vi "Prox_StateMachine.vi"(8 "error in (no error)":errorcluster) -> (0 "error out":errorcluster, 3 "aReaderName":string)   [LabVIEW 2019]
uses:
  WinSCard.dll
panel:
  out "status":string
  out "time":string
  out "pbRecvBuffer":string
  out "bATR (Answer to Reset)":string
  out "Free Memory":i32
  out "transmit":i32 format="%x"
  out "Disconnect Return":u32 format="%x"
  out "Release Context Return":u32 format="%x"
  out "Reader Return":i32 format="%x"
  out "Establish Return":u32 format="%x"
  out "Card Connect Return":u32 format="%x"
  out "Card Status Return":u32 format="%x"
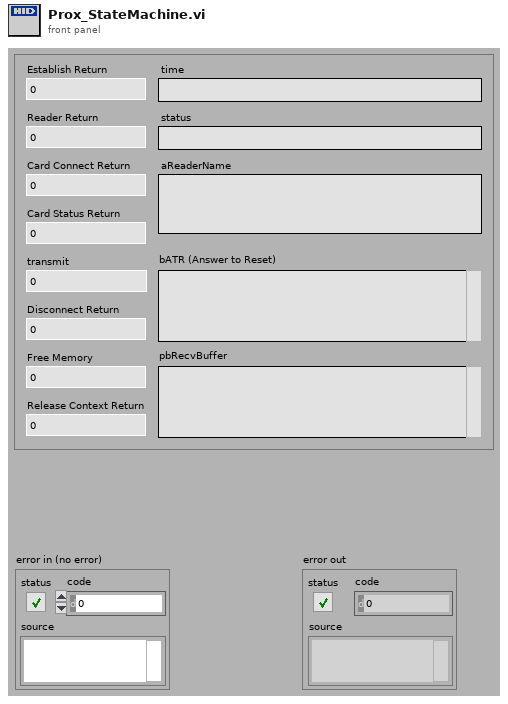
[diagram p1: front panel]
types:
  T1 = enum32{"Invalid", "Standard", "Closed", "Hidden", "Minimized", "Maximized"}
  T2 = enum32{"invalid app kind", "Development System", "Run Time System", "Student Edition", "Embedded LabVIEW", "Evaluation", "Custom"}
  T3 = enum16{"initialize", "reader present", "card connected", "card disconnected", "shutdown"}
  T4 = cluster{"Core":cluster{"Current VI Reference":refnum<vi>, "Close Panel on Exit?":bool}, "hContextHandle":u32, "hCardHandle":u32, "szReader":string, "status":enum16{"initialize", "reader present", "card connected", "card disconnected", "shutdown"}}
  T5 = cluster{"Current VI Reference":refnum<vi>, "Close Panel on Exit?":bool}
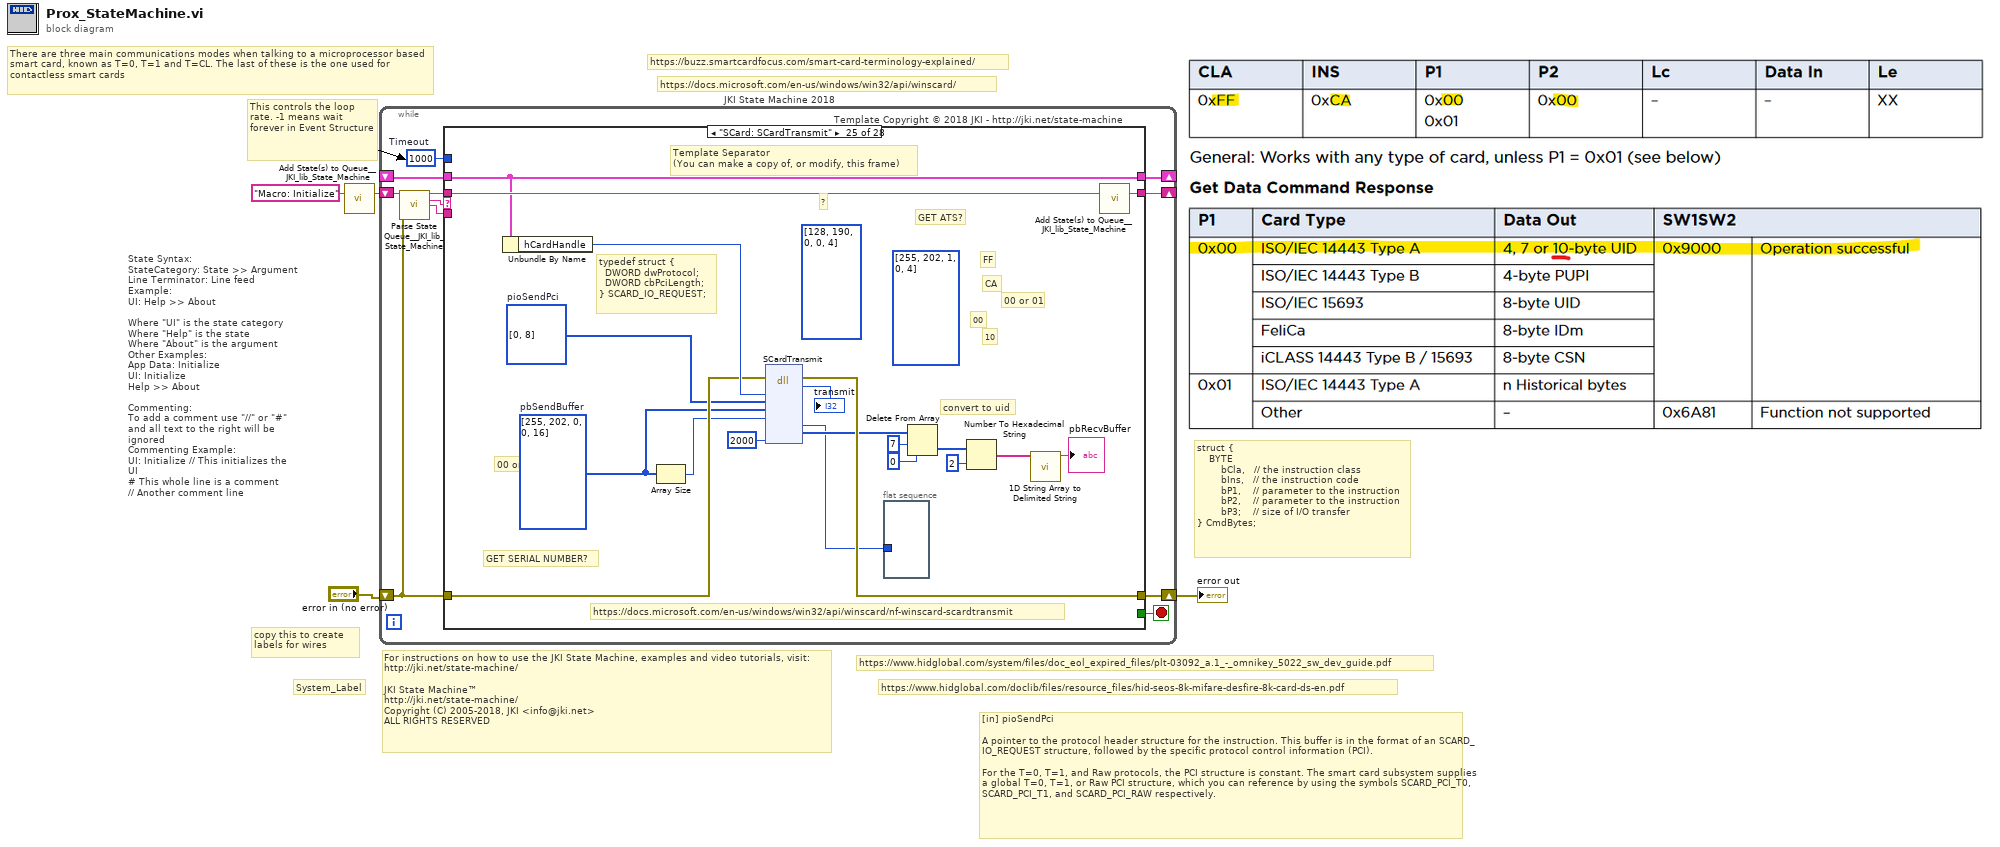
[diagram p0: block diagram]
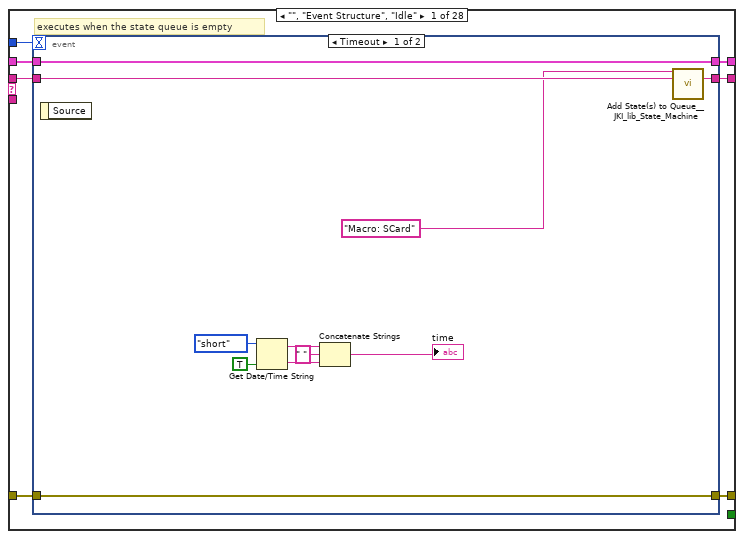
[diagram p2: hidden frame]
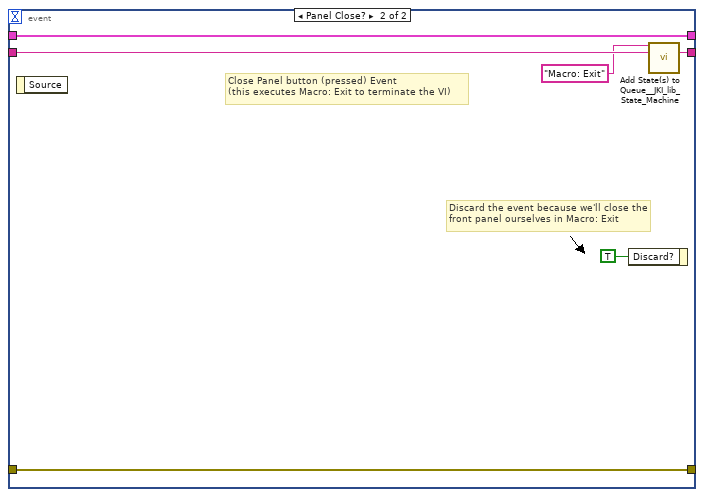
[diagram p3: hidden frame]
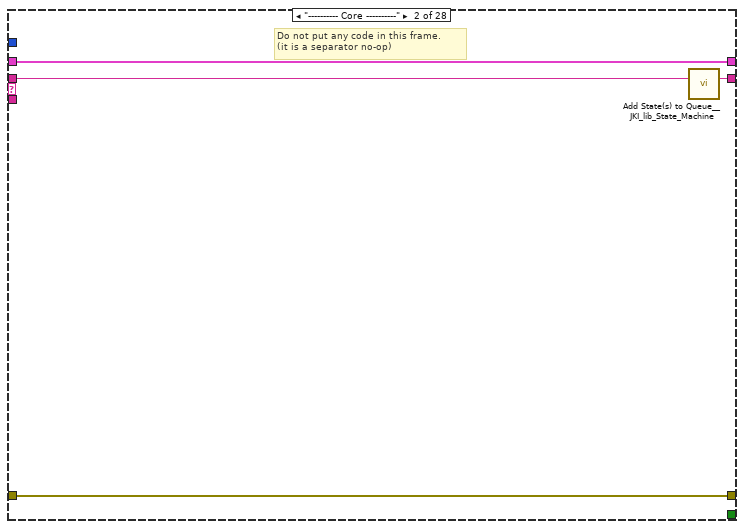
[diagram p4: hidden frame]
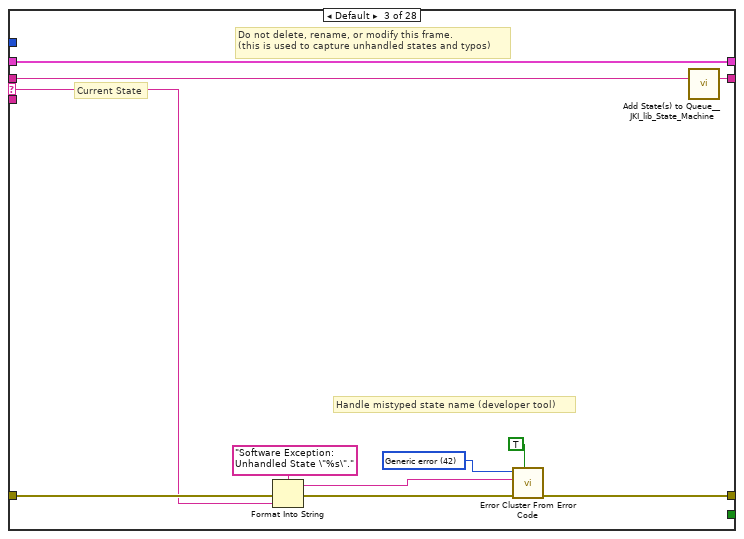
[diagram p5: hidden frame]
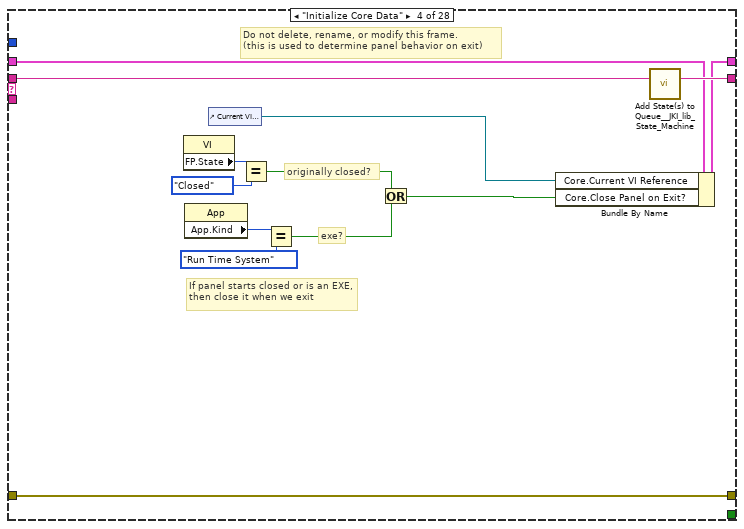
[diagram p6: hidden frame]
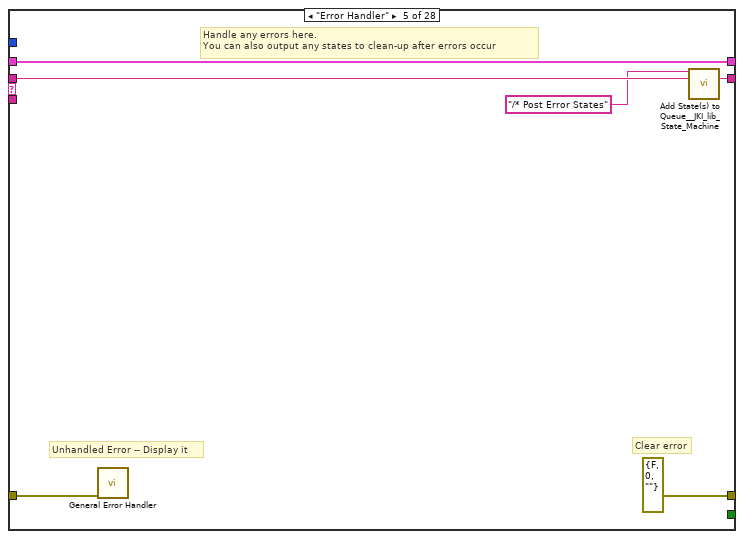
[diagram p7: hidden frame]
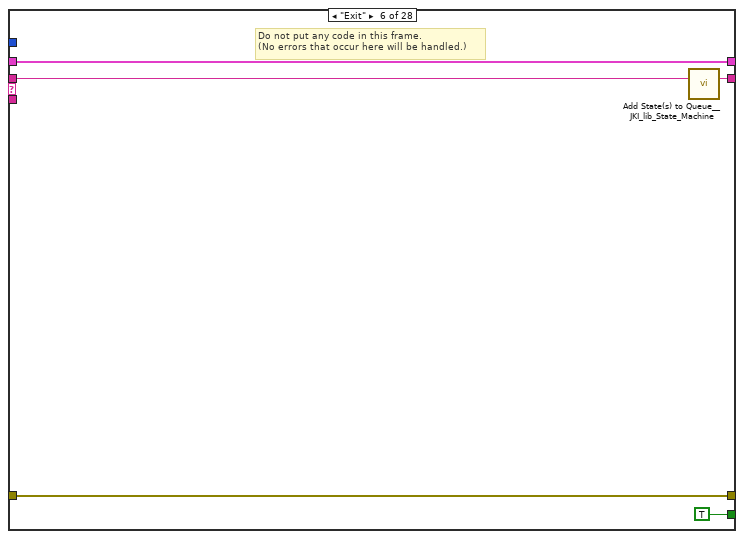
[diagram p8: hidden frame]
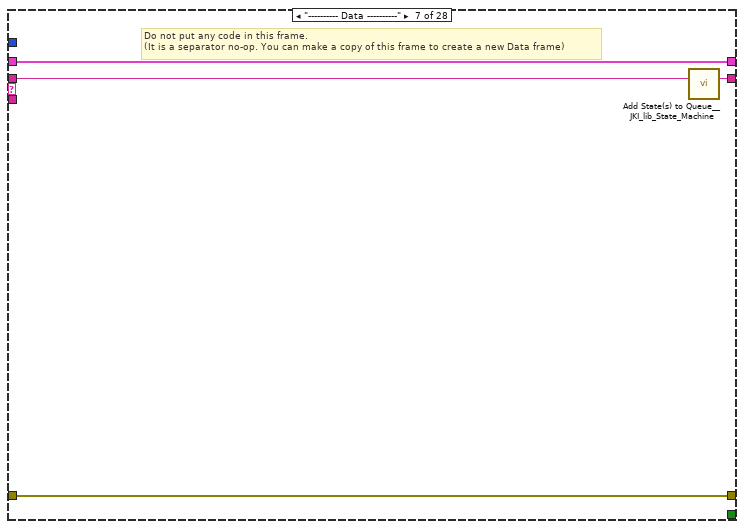
[diagram p9: hidden frame]
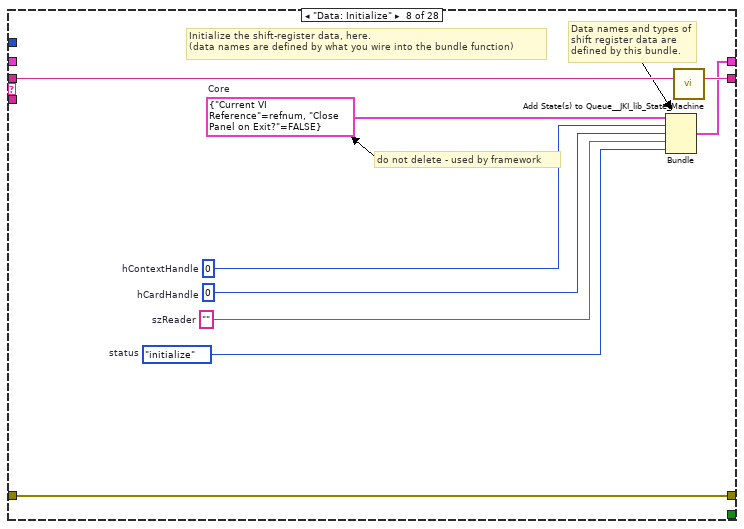
[diagram p10: hidden frame]
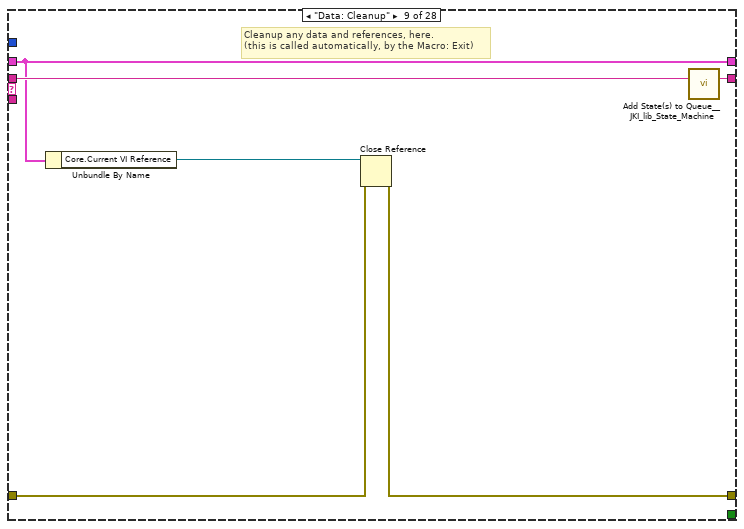
[diagram p11: hidden frame]
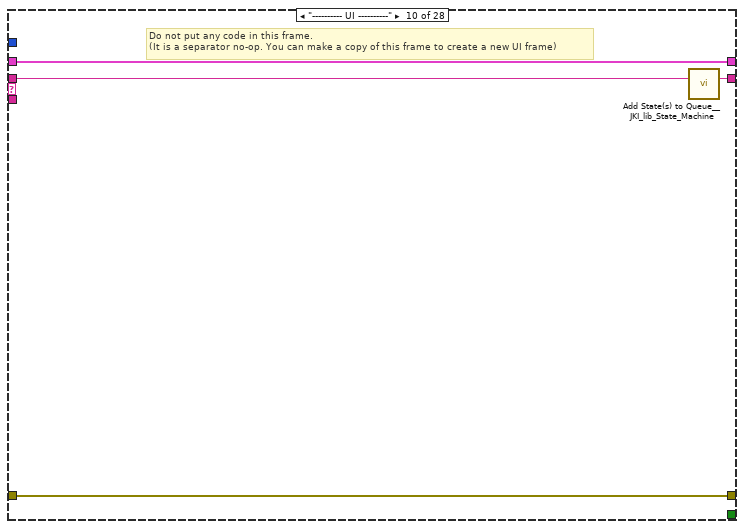
[diagram p12: hidden frame]
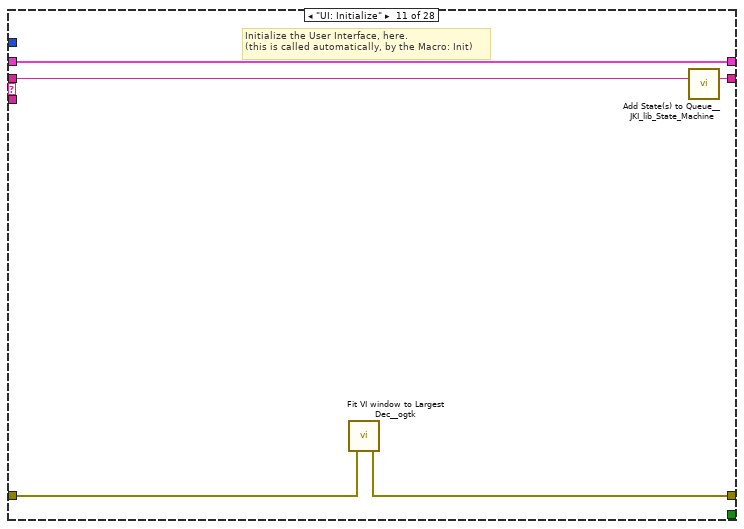
[diagram p13: hidden frame]
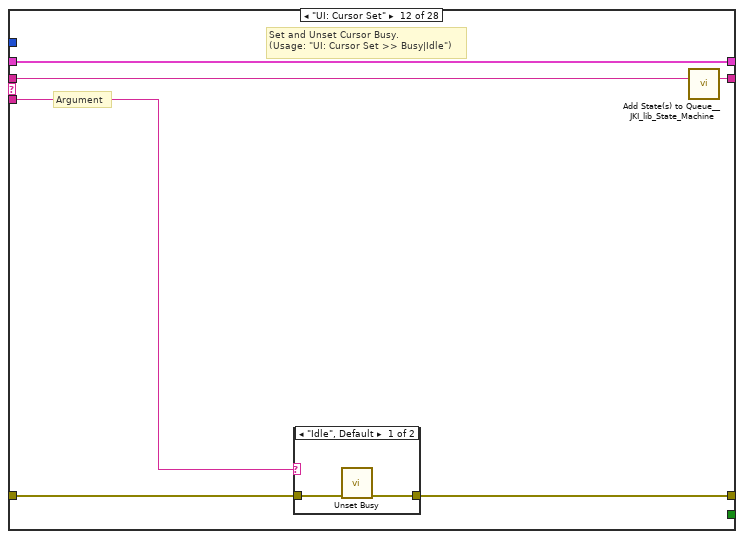
[diagram p14: hidden frame]
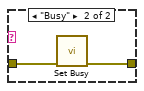
[diagram p15: hidden frame]
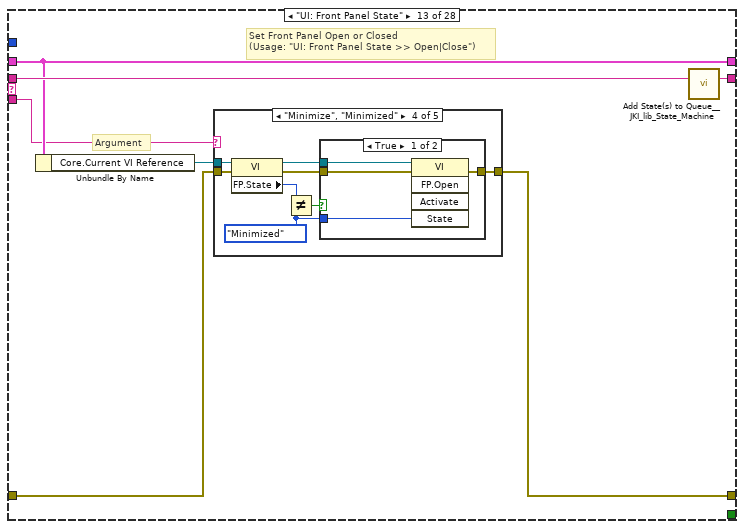
[diagram p16: hidden frame]
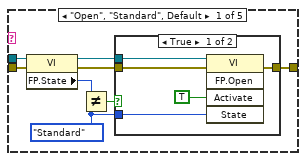
[diagram p17: hidden frame]
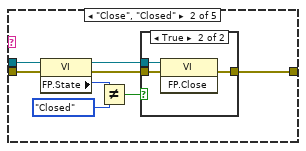
[diagram p19: hidden frame]
diagram:
  # "https://www.hidglobal.com/doclib/files/resource_files/hid-seos-8k-mifare-desfire-8k-card-ds-en.pdf"
  # "https://www.hidglobal.com/system/files/doc_eol_expired_files/plt-03092_a.1_-_omnikey_5022_sw_dev_guide.pdf"
  # "struct {\n    BYTE\n        bCla,   // the instruction class\n        bIns,   // the instruction code \n        bP1,    // parameter to the instruction\n        bP2,    // parameter to the instruction\n        bP3;    // size of I/O transfer\n} CmdBytes;"
  # "There are three main communications modes when talking to a microprocessor based smart card, known as T=0, T=1 and T=CL. The last of these is the one used for contactless smart cards"
  # "https://docs.microsoft.com/en-us/windows/win32/api/winscard/"
  # "For instructions on how to use the JKI State Machine, examples and video tutorials, visit:\nhttp://jki.net/state-machine/\n\nJKI State Machine™\nhttp://jki.net/state-machine/\nCopyright (C) 2005-2018, JKI <info@jki.net>\nALL RIGHTS RESERVED"
  # "State Syntax:\nStateCategory: State >> Argument\nLine Terminator: Line feed\nExample:\nUI: Help >> About\n\nWhere \"UI\" is the state category\nWhere \"Help\" is the state\nWhere \"About\" is the argument\nOther Examples:\nApp Data: Initialize\nUI: Initialize\nHelp >> About\n\nCommenting:\nTo add a comment use \"//\" or \"#\" and all text to the right will be ignored\nCommenting Example:\nUI: Initialize // This initializes the UI\n# This whole line is a comment\n// Another comment line"
  # "copy this to create labels for wires"
  # "This controls the loop rate. -1 means wait forever in Event Structure"
  # "System_Label"
  # "https://buzz.smartcardfocus.com/smart-card-terminology-explained/"
  # "[in] pioSendPci\n\nA pointer to the protocol header structure for the instruction. This buffer is in the format of an SCARD_IO_REQUEST structure, followed by the specific protocol control information (PCI).\n\nFor the T=0, T=1, and Raw protocols, the PCI structure is constant. The smart card subsystem supplies a global T=0, T=1, or Raw PCI structure, which you can reference by using the symbols SCARD_PCI_T0, SCARD_PCI_T1, and SCARD_PCI_RAW respectively."
  n1 = call <vilib>:"Add State(s) to Queue__JKI_lib_State_Machine.vi"("State(s) in (\"\")"="Macro: Initialize") -> ("States Out"=w4:string)  [unwired: 14 in]
  n2 = while "JKI State Machine 2018" {
    shift-right: [w8] -> _
    shift-left: _ -> [w7]
    shift-right: [w11] -> w1
    shift-left: "error in (no error)" -> [w5]
    shift-right: [w10] -> _
    shift-left: w4 -> [w12]
    stop <- w9 stop-if-true
    w6 = 1000  # Timeout
    # "Template Copyright © 2018 JKI - http://jki.net/state-machine"
    n3 = call <vilib>:"Parse State Queue__JKI_lib_State_Machine.vi"("State Queue"=w12, "Error In (no error)"=w5) -> ("Remaining States"=w14:string, "Current State"=w15:string, "Arguments"=w13:string)  [unwired: 11 in]
    n4 = case shown="\"SCard: SCardTransmit\"" w15 {
      selector: w15 -> [_ _ w44 _ _ _ _ _ _ _ _ _ _ _ _ _ _ _ _ _ _ _ _ _ _ _ _ _]
      tunnel: w14 -> [w22 w43 w48 w67 w73 w78 w82 w91 w97 w101 w106 w112 w123 w194 w198 w203 w208 _ w221 w225 w235 w241 w258 w287 w306 w314 w322 w329]
      tunnel: w13 -> [_ _ _ _ _ _ _ _ _ _ _ w107 w117 _ _ _ _ _ _ _ _ _ _ _ _ _ _ _]
      tunnel: w7 -> [w20 w40 w46 w60 w70 w76 w79 _ w92 w98 w104 w110 w119 w191 w195 w200 w205 w209 w218 w222 w228 w244 w261 w282 w303 w309 w319 w327]
      tunnel: [w19 w41 w50 w64 errorcluster {"status"=FALSE, "code"=0, "source"=""} ("error out") w75 w80 w88 w93 w99 w103 w108 w120 w192 w196 w201 w206 w210 w219 w223 w231 w242 w267 w284 w301 w311 w317 w325] -> w11
      tunnel: w5 -> [w18 w41 w49 w64 w69 w75 w80 w88 w94 w99 w102 w109 w121 w192 w196 w201 w206 w210 w219 w223 w232 w249 w266 w283 w300 w310 w316 w324]
      tunnel: [w21 w42 w47 w66 w72 w77 w81 w90 w96 w100 w105 w111 w122 w193 w197 w202 w207 w211 w220 w224 w234 w252 w270 w286 w305 w313 w321 w328] -> w10
      tunnel: [_ _ _ _ _ TRUE _ _ _ _ _ _ _ _ _ _ _ _ _ _ _ _ _ _ _ _ _ _] -> w9
      tunnel: [w17 w40 w46 w65 w70 w76 w79 w89 w92 w98 w104 w110 w119 w191 w195 w200 w205 w209 w218 w222 w229 w245 w262 w282 w303 w309 w319 w327] -> w8
      tunnel: w6 -> [w16 _ _ _ _ _ _ _ _ _ _ _ _ _ _ _ _ _ _ _ _ _ _ _ _ _ _ _]
      frame "", "Event Structure", "Idle" {
        # "executes when the state queue is empty"
        n5 = event shown="[0] Timeout" {
          selector: _ -> [_ _]
          dyn-events: _ -> [_ _]
          timeout: w16 -> [_ _]
          tunnel: w22 -> [w33 w39]
          tunnel: [w32 w38] -> w21
          tunnel: w20 -> [w30 w36]
          tunnel: [w31 w37] -> w19
          tunnel: w18 -> [w31 w37]
          tunnel: [w30 w36] -> w17
          event Timeout {
            n6 = event-data() -> ()  [unwired: 1 in, 1 out]
            n7 = Get Date/Time String(date format (0)=enum16{"short", "long", "abbreviated"}."short", want seconds? (F)=TRUE) -> (date string=w28:string, time string=w27:string)  [unwired: 1 in]
            n8 = Concatenate Strings(w28, " " ("string"), w27) -> (→"time":string)
            n9 = call <vilib>:"Add State(s) to Queue__JKI_lib_State_Machine.vi"("State(s) in Front (\"\")"="Macro: SCard" ("State(s) in Front (\"\")"), "State(s) in (\"\")"=w33) -> ("States Out"=w32:string)  [unwired: 13 in]
          }
          event Panel Close? {
            # "Discard the event because we'll close the front panel ourselves in Macro: Exit"
            # "Close Panel button (pressed) Event\n(this executes Macro: Exit to terminate the VI)"
            n10 = event-data() -> ()  [unwired: 1 in, 1 out]
            n11 = event-data("Discard?"=TRUE) -> ()  [unwired: 1 in, 1 out]
            n12 = call <vilib>:"Add State(s) to Queue__JKI_lib_State_Machine.vi"("State(s) in Front (\"\")"="Macro: Exit", "State(s) in (\"\")"=w39) -> ("States Out"=w38:string)  [unwired: 13 in]
          }
        }
      }
      frame "---------- Core ----------" {
        # "Do not put any code in this frame.\n(it is a separator no-op)"
        n13 = call <vilib>:"Add State(s) to Queue__JKI_lib_State_Machine.vi"("State(s) in (\"\")"=w43) -> ("States Out"=w42:string)  [unwired: 14 in]
      }
      frame Default {
        w53 = 42 items=["No error", "Argument error", "Memory is full", "Out of zone", "End of file", "File already open", "Generic file I/O error", "File not found", "File permission error", "Disk is full", "Duplicate path", "Too many files open", "System feature not enabled", "Resource file not found", "Cannot add resource", "Resource not found", "Image not found", "Image memory error", "Pen does not exist", "Config type invalid", "Config token not found", "Config parse error", "Config memory error", "Bad external code format", "Bad external code offset", "External code not present", "Null window", "Destroy window error", "Null menu", "Print aborted", "Bad print record", "Print driver error", "Windows error during printing", "Memory error during printing", "Print dialog error", "Generic print error", "Invalid device refnum", "Device not found", "Device parameter error", "Device unit error", "Cannot open device", "Device call aborted", "Generic error", "Cancelled by user", "Object ID too low", "Object ID too high", "Object not in heap", "Unknown heap", "Unknown object (invalid DefProc)", "Unknown object (DefProc not in table)", "Message out of range", "Invalid (null) method", "Unknown message", "Manager call not supported", "Bad address", "Network operation in progress", "Network operation timed out", "Connection is busy", "Network attribute not supported", "Network error", "Address in use", "System out of memory", "Connection aborted", "Connection refused", "Not connected", "Already connected", "Connection closed", "Initialization error (interapplication manager)", "Bad occurrence", "Wait on unbound occurrence handler", "Occurrence queue overflow", "Datalog type conflict", "Unused", "Unrecognized type (interapplication manager)", "Memory corrupt", "Failed to make temporary DLL", "Old CIN version", "Drag socket not found", "Failed to load drop-object", "Failed to register OLE object", "Failed to release OLE object", "Format specifier type mismatch", "Unknown format specifier", "Too few format specifiers", "Too many format specifiers", "Scan failed", "Newer CIN version", "Error converting to variant", "Runtime menu error", "Password tampered", "Variant attribute not found", "Incompatible variant data type", "Event data is not available", "Event Store is not present", "Occurrence is not found", "Event Queue is not created", "Event info is not available", "Refnum passed is NULL", "Error retrieving Class GUID", "Error retrieving CoClass GUID", "Error retrieving TypeLib GUID.", "Bad built application magic bytes.", "Specific driver is different from the specific driver associated with the Logical Name.", "There is no session opened to the class driver.", "Max Error", "MAX - Error with config objects", "MAX - Error loading configuration", "MAX - Group not supported"]
        # "Current State"
        # "Do not delete, rename, or modify this frame.\n(this is used to capture unhandled states and typos)"
        # "Handle mistyped state name (developer tool)"
        n14 = Format Into String(format string="Software Exception: Unhandled State \"%s\"." ("message"), error in=w49, w44) -> (resulting string=w52:string, error out=w51:errorcluster)  [unwired: 1 in]
        n15 = call <vilib>:"Error Cluster From Error Code.vi"("show call chain? (False)"=TRUE, "error in (no error)"=w51, "error message (\"\")"=w52, "error code (0)"=w53) -> ("error out"=w50:errorcluster)  [unwired: 5 in]
        n16 = call <vilib>:"Add State(s) to Queue__JKI_lib_State_Machine.vi"("State(s) in (\"\")"=w48) -> ("States Out"=w47:string)  [unwired: 14 in]
      }
      frame "Initialize Core Data" {
        # "Do not delete, rename, or modify this frame.\n(this is used to determine panel behavior on exit)"
        # "originally closed?"
        # "exe?"
        # "If panel starts closed or is an EXE, then close it when we exit"
        n17 = property class="VI"() -> ("FP.State"=w57:T1)  [unwired: 2 in, 2 out]
        n18 = property class="App"() -> ("App.Kind"=w63:T2)  [unwired: 2 in, 2 out]
        n19 = control-ref of="Current VI Reference"() -> (w58:refnum<vi>)
        n20 = Equal?(x=w57, y=T1."Closed" ("Front Panel Window:State")) -> (x = y?=w55:bool)
        n21 = Equal?(x=w63, y=T2."Run Time System" ("Application:Kind")) -> (x = y?=w61:bool)
        n22 = Or(x=w55, y=w61) -> (x .or. y?=w59:bool)
        n23 = Bundle By Name(cluster=w60, "Core.Current VI Reference"=w58, "Core.Close Panel on Exit?"=w59) -> (w65:T4)
        n24 = call <vilib>:"Add State(s) to Queue__JKI_lib_State_Machine.vi"("State(s) in (\"\")"=w67) -> ("States Out"=w66:string)  [unwired: 14 in]
      }
      frame "Error Handler" {
        # "Unhandled Error -- Display it"
        # "Handle any errors here.\nYou can also output any states to clean-up after errors occur"
        # "Clear error"
        n25 = call <vilib>:"General Error Handler.vi"("error in (no error)"=w69) -> ()  [unwired: 10 in, 5 out]
        n26 = call <vilib>:"Add State(s) to Queue__JKI_lib_State_Machine.vi"("State(s) in Front (\"\")"="/* Post Error States", "State(s) in (\"\")"=w73) -> ("States Out"=w72:string)  [unwired: 13 in]
      }
      frame "Exit" {
        # "Do not put any code in this frame.\n(No errors that occur here will be handled.)"
        n27 = call <vilib>:"Add State(s) to Queue__JKI_lib_State_Machine.vi"("State(s) in (\"\")"=w78) -> ("States Out"=w77:string)  [unwired: 14 in]
      }
      frame "---------- Data ----------" {
        # "Do not put any code in this frame.\n(It is a separator no-op. You can make a copy of this frame to create a new Data frame)"
        n28 = call <vilib>:"Add State(s) to Queue__JKI_lib_State_Machine.vi"("State(s) in (\"\")"=w82) -> ("States Out"=w81:string)  [unwired: 14 in]
      }
      frame "Data: Initialize" {
        w83 = T3."initialize"  # status
        w84 = ""  # szReader
        w85 = u32 0  # hCardHandle
        w86 = u32 0  # hContextHandle
        w87 = T5 {"Current VI Reference"=refnum, "Close Panel on Exit?"=FALSE}  # Core
        # "do not delete - used by framework"
        # "Data names and types of shift register data are defined by this bundle."
        # "Initialize the shift-register data, here.\n(data names are defined by what you wire into the bundle function)"
        n29 = Bundle("Core"=w87, "hContextHandle"=w86, "hCardHandle"=w85, "szReader"=w84, "status"=w83) -> (w89:T4)  [unwired: 1 in]
        n30 = call <vilib>:"Add State(s) to Queue__JKI_lib_State_Machine.vi"("State(s) in (\"\")"=w91) -> ("States Out"=w90:string)  [unwired: 14 in]
      }
      frame "Data: Cleanup" {
        # "Cleanup any data and references, here.\n(this is called automatically, by the Macro: Exit)"
        n31 = Unbundle By Name(w92) -> ("Core.Current VI Reference"=w95:refnum<vi>)
        n32 = Close Reference(reference=w95, error in (no error)=w94) -> (error out=w93:errorcluster)
        n33 = call <vilib>:"Add State(s) to Queue__JKI_lib_State_Machine.vi"("State(s) in (\"\")"=w97) -> ("States Out"=w96:string)  [unwired: 14 in]
      }
      frame "---------- UI ----------" {
        # "Do not put any code in this frame.\n(It is a separator no-op. You can make a copy of this frame to create a new UI frame)"
        n34 = call <vilib>:"Add State(s) to Queue__JKI_lib_State_Machine.vi"("State(s) in (\"\")"=w101) -> ("States Out"=w100:string)  [unwired: 14 in]
      }
      frame "UI: Initialize" {
        # "Initialize the User Interface, here.\n(this is called automatically, by the Macro: Init)"
        n35 = call <userlib>:"Fit VI window to Largest Dec__ogtk.vi"("error in (no error)"=w102) -> ("error out"=w103:errorcluster)  [unwired: 5 in, 1 out]
        n36 = call <vilib>:"Add State(s) to Queue__JKI_lib_State_Machine.vi"("State(s) in (\"\")"=w106) -> ("States Out"=w105:string)  [unwired: 14 in]
      }
      frame "UI: Cursor Set" {
        # "Argument"
        # "Set and Unset Cursor Busy.\n(Usage: \"UI: Cursor Set >> Busy|Idle\")"
        n37 = case shown="\"Idle\", Default" w107 {
          tunnel: w109 -> [w114 w116]
          tunnel: [w113 w115] -> w108
          frame "Idle", Default {
            n38 = call <vilib>:"Unset Busy.vi"("error in (no error)"=w114) -> ("error out"=w113:errorcluster)  [unwired: 10 in]
          }
          frame "Busy" {
            n39 = call <vilib>:"Set Busy.vi"("error in (no error)"=w116) -> ("error out"=w115:errorcluster)  [unwired: 9 in, 1 out]
          }
        }
        n40 = call <vilib>:"Add State(s) to Queue__JKI_lib_State_Machine.vi"("State(s) in (\"\")"=w112) -> ("States Out"=w111:string)  [unwired: 14 in]
      }
      frame "UI: Front Panel State" {
        # "Argument"
        # "Set Front Panel Open or Closed\n(Usage: \"UI: Front Panel State >> Open|Close\")"
        n41 = Unbundle By Name(w119) -> ("Core.Current VI Reference"=w118:refnum<vi>)
        n42 = case shown="\"Minimize\", \"Minimized\"" w117 {
          tunnel: w121 -> [w129 w144 w155 w168 w181]
          tunnel: [w131 w145 w157 w170 w183] -> w120
          tunnel: w118 -> [w130 w142 w156 w169 w182]
          frame "Open", "Standard", Default {
            w124 = T1."Standard" ("State")
            n43 = property class="VI"(reference=w130, error in=w129) -> (reference out=w127:refnum<vi>, error out=w128:errorcluster, "FP.State"=w126:T1)
            n44 = Not Equal?(x=w126, y=w124) -> (x != y?=w125:bool)
            n45 = case shown="True" w125 {
              tunnel: [w135 w137] -> w131
              tunnel: w128 -> [w134 w137]
              tunnel: w127 -> [w133 _]
              tunnel: w124 -> [w132 _]
              frame True {
                n46 = invoke class="VI" method="FP.Open"(reference=w133, error in=w134, "Activate"=TRUE, "State"=w132) -> (error out=w135:errorcluster)  [unwired: 1 in, 4 out]
              }
              frame False {
              }
            }
          }
          frame "Close", "Closed" {
            n47 = property class="VI"(reference=w142, error in=w144) -> (reference out=w141:refnum<vi>, error out=w143:errorcluster, "FP.State"=w139:T1)
            n48 = Not Equal?(x=w139, y=T1."Closed" ("Front Panel Window:State")) -> (x != y?=w138:bool)
            n49 = case shown="True" w138 {
              tunnel: [w146 w149] -> w145
              tunnel: w143 -> [w146 w148]
              tunnel: w141 -> [_ w147]
              frame False {
              }
              frame True {
                n50 = invoke class="VI" method="FP.Close"(reference=w147, error in=w148) -> (error out=w149:errorcluster)  [unwired: 1 in, 2 out]
              }
            }
          }
          frame "Hidden", "Hide" {
            w150 = T1."Hidden" ("State")
            n51 = property class="VI"(reference=w156, error in=w155) -> (reference out=w153:refnum<vi>, error out=w154:errorcluster, "FP.State"=w152:T1)
            n52 = Not Equal?(x=w152, y=w150) -> (x != y?=w151:bool)
            n53 = case shown="True" w151 {
              tunnel: [w161 w162] -> w157
              tunnel: w154 -> [w160 w162]
              tunnel: w153 -> [w159 _]
              tunnel: w150 -> [w158 _]
              frame True {
                n54 = invoke class="VI" method="FP.Open"(reference=w159, error in=w160, "State"=w158) -> (error out=w161:errorcluster)  [unwired: 2 in, 4 out]
              }
              frame False {
              }
            }
          }
          frame "Minimize", "Minimized" {
            w163 = T1."Minimized" ("State")
            n55 = property class="VI"(reference=w169, error in=w168) -> (reference out=w166:refnum<vi>, error out=w167:errorcluster, "FP.State"=w165:T1)
            n56 = Not Equal?(x=w165, y=w163) -> (x != y?=w164:bool)
            n57 = case shown="True" w164 {
              tunnel: [w174 w175] -> w170
              tunnel: w167 -> [w173 w175]
              tunnel: w166 -> [w172 _]
              tunnel: w163 -> [w171 _]
              frame True {
                n58 = invoke class="VI" method="FP.Open"(reference=w172, error in=w173, "State"=w171) -> (error out=w174:errorcluster)  [unwired: 2 in, 4 out]
              }
              frame False {
              }
            }
          }
          frame "Maximize", "Maximized" {
            w176 = T1."Maximized" ("State")
            n59 = property class="VI"(reference=w182, error in=w181) -> (reference out=w179:refnum<vi>, error out=w180:errorcluster, "FP.State"=w178:T1)
            n60 = Not Equal?(x=w178, y=w176) -> (x != y?=w177:bool)
            n61 = case shown="True" w177 {
              tunnel: [w187 w188] -> w183
              tunnel: w180 -> [w186 w188]
              tunnel: w179 -> [w185 _]
              tunnel: w176 -> [w184 _]
              frame True {
                n62 = invoke class="VI" method="FP.Open"(reference=w185, error in=w186, "State"=w184) -> (error out=w187:errorcluster)  [unwired: 2 in, 4 out]
              }
              frame False {
              }
            }
          }
        }
        n63 = call <vilib>:"Add State(s) to Queue__JKI_lib_State_Machine.vi"("State(s) in (\"\")"=w123) -> ("States Out"=w122:string)  [unwired: 14 in]
      }
      frame "UI: Update Status" {
        # "Do not put any code in this frame.\n(It is a separator no-op. You can make a copy of this frame to create a new UI frame)"
        n64 = Unbundle By Name(w191) -> ("status"=w190:T3)
        n65 = Format Into String(w190) -> (resulting string=→"status":string)  [unwired: 3 in, 1 out]
        n66 = call <vilib>:"Add State(s) to Queue__JKI_lib_State_Machine.vi"("State(s) in (\"\")"=w194) -> ("States Out"=w193:string)  [unwired: 14 in]
      }
      frame "---------- Macro ----------" {
        # "Do not put any code in this frame.\n(It is a separator no-op. You can make a copy of this frame to create a new Macro frame)"
        n67 = call <vilib>:"Add State(s) to Queue__JKI_lib_State_Machine.vi"("State(s) in (\"\")"=w198) -> ("States Out"=w197:string)  [unwired: 14 in]
      }
      frame "Macro: Initialize" {
        w199 = "Data: Initialize\nInitialize Core Data\nUI: Initialize\nUI: Front Panel State >> Open"  # Data: Initialize Initialize Core Data UI: Initialize UI: Front Panel State >> Open
        # "Initialization Macro\n(This is called once, when the VI starts)"
        n68 = call <vilib>:"Add State(s) to Queue__JKI_lib_State_Machine.vi"("State(s) in Front (\"\")"=w199, "State(s) in (\"\")"=w203) -> ("States Out"=w202:string)  [unwired: 13 in]
      }
      frame "Macro: SCard" {
        # "Do not put any code in this frame.\n(It is a separator no-op. You can make a copy of this frame to create a new Macro frame)"
        n69 = call <vilib>:"Add State(s) to Queue__JKI_lib_State_Machine.vi"("State(s) in Front (\"\")"="SCard: SCardEstablishContext\nUI: Update Status\nSCard: SCardListReadersA\nUI: Update Status\nSCard: SCardConnectA\nUI: Update Status\nSCard: SCardStatusA\nUI: Update Status\nSCard: SCardTransmit\nUI: Update Status\nSCard: SCardDisconnect\nUI: Update Status\nSCard: SCardFreeMemory\nUI: Update Status\nSCard: SCardReleaseContext\nUI: Update Status" ("State(s) in Front (\"\")"), "State(s) in (\"\")"=w208) -> ("States Out"=w207:string)  [unwired: 13 in]
      }
      frame "Macro: Abort" {
        # "Do not put any code in this frame.\n(It is a separator no-op. You can make a copy of this frame to create a new Macro frame)"
        n70 = call <vilib>:"Add State(s) to Queue__JKI_lib_State_Machine.vi"() -> ("States Out"=w211:string)  [unwired: 15 in]
      }
      frame "Macro: Exit" {
        # "Exit Macro\n(This is called once, when the VI exits)"
        n71 = Unbundle By Name(w218) -> ("Core.Close Panel on Exit?"=w217:bool)
        n72 = Select(t="UI: Front Panel State >> Close", s=w217, f="") -> (s? t:f=w214:string)
        n73 = call <vilib>:"Add State(s) to Queue__JKI_lib_State_Machine.vi"("State(s) in (\"\")"=w214, "State(s) at Back (\"\")"="Data: Cleanup\nExit") -> ("States Out"=w212:string)  [unwired: 13 in]
        n74 = call <vilib>:"Add State(s) to Queue__JKI_lib_State_Machine.vi"("State(s) in Front (\"\")"=w212, "State(s) in (\"\")"=w221) -> ("States Out"=w220:string)  [unwired: 13 in]
      }
      frame "---------- SCard ----------" {
        # "Template Separator\n(You can make a copy of, or modify, this frame)"
        n75 = call <vilib>:"Add State(s) to Queue__JKI_lib_State_Machine.vi"("State(s) in (\"\")"=w225) -> ("States Out"=w224:string)  [unwired: 14 in]
      }
      frame "SCard: SCardEstablishContext" {
        w226 = u32 0
        # "Your code here.\n(You can make a copy of, or modify, this frame)"
        n76 = dll-call lib="winscard.dll" fn="SCardEstablishContext"(error in=w232, "SCARD_SCOPE_USER"=u32 0, "NULL1"=w226, "NULL2"=w226) -> (error out=w231:errorcluster, "return type"=→"Establish Return":u32, "hContextHandle"=w230:u32)  [unwired: 5 in, 2 out]
        n77 = Bundle By Name(cluster=w228, "hContextHandle"=w230) -> (w229:T4)
        n78 = call <vilib>:"Add State(s) to Queue__JKI_lib_State_Machine.vi"("State(s) in (\"\")"=w235) -> ("States Out"=w234:string)  [unwired: 14 in]
      }
      frame "SCard: SCardListReadersA" {
        # "Your code here.\n(You can make a copy of, or modify, this frame)"
        n79 = Unbundle By Name(w244) -> ("status"=w237:T3, "hContextHandle"=w248:u32)
        n80 = dll-call lib="winscard.dll" fn="SCardListReadersA"(error in=w249, "hContextHandle"=w248, "NULL3"=0, "dwReaderListLength"=u32 100) -> (error out=w242:errorcluster, "lresult"=w240:i32, "hContextHandle"=w246:u32, "bReaderListBuffer"=w247:u8[])  [unwired: 3 in, 3 out]
        "Reader Return" <- w240
        n81 = Byte Array To String(unsigned byte array=w247) -> (string=w243:string)
        n82 = Equal To 0?(x=w240) -> (x = 0?=w239:bool)
        n83 = Select(t=T3."reader present" ("status"), s=w239, f=w237) -> (s? t:f=w238:T3)
        n84 = Bundle By Name(cluster=w244, "status"=w238, "hContextHandle"=w246, "szReader"=w243) -> (w245:T4)
        n85 = call <vilib>:"Add State(s) to Queue__JKI_lib_State_Machine.vi"("State(s) in (\"\")"=w241) -> ("States Out"=w252:string)  [unwired: 14 in]
      }
      frame "SCard: SCardConnectA" {
        # "Template Separator\n(You can make a copy of, or modify, this frame)"
        n86 = Unbundle By Name(w261) -> ("hContextHandle"=w265:u32, "szReader"=w264:string)  [unwired: 1 out]
        n87 = dll-call lib="winscard.dll" fn="SCardConnectA"(error in=w266, "hContextHandle"=w265, "szReader"=w264, "SCARD_SHARE_SHARED"=u32 2, "SCARD_PROTOCOL_T0"=u32 3 ("SCARD_SHARE_SHARED")) -> (error out=w267:errorcluster, "lreturn"=w255:u32, "SCARD_PROTOCOL_T0"=w259:u32, "hCardHandle"=w263:u32, "dwAP"=w260:i32)  [unwired: 5 in, 3 out]
        "Card Connect Return" <- w255
        n88 = flat-sequence {
          tunnel: w260 -> [_]
          tunnel: w259 -> [_]
          frame #0 {
          }
        }
        n89 = Equal To 0?(x=w255) -> (x = 0?=w257:bool)
        n90 = Select(t=T3."card connected" ("status"), s=w257, f=T3."card disconnected" ("status")) -> (s? t:f=w254:T3)
        n91 = Bundle By Name(cluster=w261, "status"=w254, "hCardHandle"=w263) -> (w262:T4)
        n92 = call <vilib>:"Add State(s) to Queue__JKI_lib_State_Machine.vi"("State(s) in (\"\")"=w258) -> ("States Out"=w270:string)  [unwired: 14 in]
      }
      frame "SCard: SCardStatusA" {
        # "Template Separator\n(You can make a copy of, or modify, this frame)"
        n93 = Unbundle By Name(w282) -> ("hCardHandle"=w281:u32, "szReader"=w280:string)
        n94 = dll-call lib="winscard.dll" fn="SCardStatusA"(error in=w283, "hCardHandle"=w281, "aReaderName"=w280, "dwATRLEN"=u32 50) -> (error out=w284:errorcluster, "lreturn"=→"Card Status Return":u32, "aReaderName"=→"aReaderName":string, "dwReaderNamelen"=w275:u32, "dwstate"=w277:u32, "Protocol"=w276:u32, "bATR"=w274:u8[])  [unwired: 3 in, 6 out]
        n95 = Number To Hexadecimal String(1:i16 2 ("width (-)"), 2:w274) -> (0:w273:string[])
        n96 = call <vilib>:"1D String Array to Delimited String.vi"("string array"=w273) -> ("delimited string"=→"bATR (Answer to Reset)":string)  [unwired: 10 in]
        n97 = flat-sequence {
          tunnel: w277 -> [_]
          tunnel: w276 -> [_]
          tunnel: w275 -> [_]
          frame #0 {
          }
        }
        n98 = call <vilib>:"Add State(s) to Queue__JKI_lib_State_Machine.vi"("State(s) in (\"\")"=w287) -> ("States Out"=w286:string)  [unwired: 14 in]
      }
      frame "SCard: SCardTransmit" {
        (unwired) u8[] [255, 202, 1, 0, 4]
        (unwired) u8[] [128, 190, 0, 0, 4]
        w298 = u8[] [255, 202, 0, 0, 16]  # pbSendBuffer
        w297 = u32[] [0, 8]  # pioSendPci
        # "convert to uid"
        # "00 or 01"
        # "10"
        # "00"
        # "00 or 01"
        # "CA"
        # "FF"
        # "typedef struct {\n  DWORD dwProtocol;\n  DWORD cbPciLength;\n} SCARD_IO_REQUEST;"
        # "https://docs.microsoft.com/en-us/windows/win32/api/winscard/nf-winscard-scardtransmit"
        # "or"
        # "GET ATS?"
        # "?"
        # "GET SERIAL NUMBER?"
        # "Template Separator\n(You can make a copy of, or modify, this frame)"
        n99 = Unbundle By Name(w303) -> ("hCardHandle"=w302:u32)
        n100 = Array Size(array=w298) -> (size(s)=w299:i32)
        n101 = dll-call lib="winscard.dll" fn="SCardTransmit"(error in=w300, "hCardHandle"=w302, "pioSendPci"=w297, "pbSendBuffer"=w298, "cbSendLen"=w299, "pcbRecvLen"=u32 2000) -> (error out=w301:errorcluster, "lreturn2"=→"transmit":i32, "pioRecvPci"=w292:u32, "pbRecvBuffer"=w294:u8[])  [unwired: 9 in, 1 out]
        n102 = flat-sequence {
          tunnel: w292 -> [_]
          frame #0 {
          }
        }
        n103 = Delete From Array(array=w294, length=7, index=0) -> (deleted portion=w291:u8[])  [unwired: 1 out]
        n104 = Number To Hexadecimal String(1:i16 2 ("width (-)"), 2:w291) -> (0:w290:string[])
        n105 = call <vilib>:"1D String Array to Delimited String.vi"("string array"=w290) -> ("delimited string"=→"pbRecvBuffer":string)  [unwired: 10 in]
        n106 = call <vilib>:"Add State(s) to Queue__JKI_lib_State_Machine.vi"("State(s) in (\"\")"=w306) -> ("States Out"=w305:string)  [unwired: 14 in]
      }
      frame "SCard: SCardDisconnect" {
        # "Template Separator\n(You can make a copy of, or modify, this frame)"
        n107 = Unbundle By Name(w309) -> ("hCardHandle"=w308:u32)
        n108 = dll-call lib="winscard.dll" fn="SCardDisconnect"(error in=w310, "hCardHandle"=w308, "dwDisposition"=u32 3 ("dwATRLEN")) -> (error out=w311:errorcluster, "lreturn"=→"Disconnect Return":u32)  [unwired: 4 in, 1 out]
        n109 = call <vilib>:"Add State(s) to Queue__JKI_lib_State_Machine.vi"("State(s) in (\"\")"=w314) -> ("States Out"=w313:string)  [unwired: 14 in]
      }
      frame "SCard: SCardFreeMemory" {
        # "Template Separator\n(You can make a copy of, or modify, this frame)"
        n110 = Unbundle By Name(w319) -> ("hContextHandle"=w318:u32)
        n111 = dll-call lib="winscard.dll" fn="SCardFreeMemory"(error in=w316, "hContextHandle"=w318, "bReaderListBuffer"=0) -> (error out=w317:errorcluster, "lreturn2"=→"Free Memory":i32)  [unwired: 4 in, 1 out]
        n112 = call <vilib>:"Add State(s) to Queue__JKI_lib_State_Machine.vi"("State(s) in (\"\")"=w322) -> ("States Out"=w321:string)  [unwired: 14 in]
      }
      frame "SCard: SCardReleaseContext" {
        # "Template Separator\n(You can make a copy of, or modify, this frame)"
        n113 = Unbundle By Name(w327) -> ("hContextHandle"=w326:u32)
        n114 = dll-call lib="winscard.dll" fn="SCardReleaseContext"(error in=w324, "contextHandle"=w326) -> (error out=w325:errorcluster, "return type"=→"Release Context Return":u32)  [unwired: 3 in, 1 out]
        n115 = call <vilib>:"Add State(s) to Queue__JKI_lib_State_Machine.vi"("State(s) in (\"\")"=w329) -> ("States Out"=w328:string)  [unwired: 14 in]
      }
    }
  }
  "error out" <- w1
